vi "Transmission Ratio.vi"(9 "Transmission Speed Out (rad/s)":sgl, 10 "Gear":sgl, 11 "Transmission Torque In (N-m)":sgl) -> (1 "Transmission Speed In (rad/s)":sgl, 2 "Transmission Torque Out (N-m)":sgl)   [LabVIEW 2016, in "NI-PCG Vehicle Model.lvlib"]
uses:
  NI-PCG Vehicle Model.lvlib
  Globals/Parameters.vi
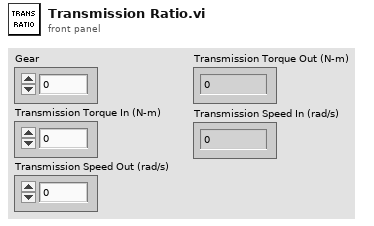
[diagram p1: front panel]
types:
  T1 = typedef "NI-PCG Vehicle Model.lvlib/Engine Parameters.ctl" = cluster{"Ambient Parameters":cluster{"Temperature (K)":sgl, "Pressure (Pa)":sgl}, "Air Parameters":cluster{"R (Ideal Gas Constant)":sgl, "Molecular Weight":sgl, "Cp (Specific Heat Constant)":sgl, "Density (kg/m^3)":sgl, "Stoichiometric A/F Ratio":sgl}, "Engine Geometry Parameters":cluster{"Cylinder Volume (l)":sgl, "J (Rotational Moment of Inertia)":sgl, "Minimuim Engine Speed":sgl, "Maximum Engine Speed":sgl, "Intake Manifold Volume (l)":sgl}, "Volumetric Efficiency Map":cluster{"MAP":sgl[], "RPM":sgl[], "Table":sgl[][]}, "Fuel LHV (J/kg)":sgl, "Combustion Efficiency Map":cluster{"Spark Timing (deg BTDC))":sgl[], "Engine Speed (RPM)":sgl[], "Combustion Efficiency":sgl[][]}, "Thermodynamic Efficiency":sgl}
  T2 = typedef "NI-PCG Vehicle Model.lvlib/Transmission Parameters.ctl" = cluster{"Final Drive Ratio":sgl, "Transmission Gear Ratios":cluster{"Gears":sgl[], "Gear Ratios":sgl[]}, "Torque Converter Map":cluster{"Speed Ratio":sgl[], "K Factor":sgl[], "Torque Ratio":sgl[]}, "Upshift Throttle":sgl[], "Downshift Throttle":sgl[], "Upshift Table":sgl[][], "Downshift Table":sgl[][], "Wait Time":u8}
  T3 = typedef "NI-PCG Vehicle Model.lvlib/Vehicle Parameters.ctl" = cluster{"Vehicle Mass (kg)":sgl, "Vehicle Cd":sgl, "Vehicle Frontal Area (m^2)":sgl, "Wheel Radius (m)":sgl, "Wheel Rolling Resistance":sgl}
  T4 = cluster{"Engine Parameters":T1, "Transmission Parameters":T2, "Vehicle Parameters":T3}
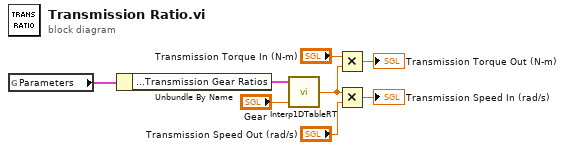
[diagram p0: block diagram]
diagram:
  n1 = global read "Parameters.vi" "Parameters"() -> (w1:T4)
  n2 = Unbundle By Name(w1) -> ("Transmission Parameters.Transmission Gear Ratios"=w8:cluster{"Gears":sgl[], "Gear Ratios":sgl[]})
  n3 = call <vilib>:"Interp1DTableRT.vi"("X"="Gear", "1DTable"=w8) -> ("Y"=w4:sgl)  [unwired: 1 in]
  n4 = Multiply(x="Transmission Torque In (N-m)", y=w4) -> (x*y=→"Transmission Torque Out (N-m)":sgl)
  n5 = Multiply(x=w4, y="Transmission Speed Out (rad/s)") -> (x*y=→"Transmission Speed In (rad/s)":sgl)
